vi "Apply Savitzky Golay Filter.vi"(0 "Waveform Graph":waveform(dbl)[](array[waveform])=[{"t0"=timestamp(0 s since 1904-01-01), "dt"=1.9999999999999998e-05, "Y"=array[781097 elements]}, {"t0"=timestamp(0 s since 1904-01-01), "dt"=1.9999999999999998e-05, "Y"=array[781097 elements]}], 2 "Savitzksky-Golay param":T1={"Sidepoints (M)"=20, "Filter Order"=5} {"Filter Order" scale=0.0..10.0; "Sidepoints (M)" scale=0.0..10.0}, 5 "error in (no error)":errorcluster) -> (14 "Waveform(s) out":waveform(dbl)[](array[waveform]), 19 "error out":errorcluster)   [LabVIEW 2019, in "Fcurve.lvclass"]
doc: "Decimates a waveform ptbypt with given parameters. Sidepoint (M), ordered polynomial refers to the polynomial order fitting parameter. \nNote: # of channels set to 1, can be configured to filter all channels when needed\n\nInput:\nWaveform graphs: [0] Deflection (V), [1] Zposition (V)\n\nOutput: \nWfms ([0] deflection) : [0] Filtered_Deflection (V). [1] Zposition (V)"
uses:
  Fcurve.lvclass
  <vilib>/ptbypt/NI_PtbyPt.lvlib
panel:
  out "Wfms ([0]deflection)":dbl[][](array[numeric])
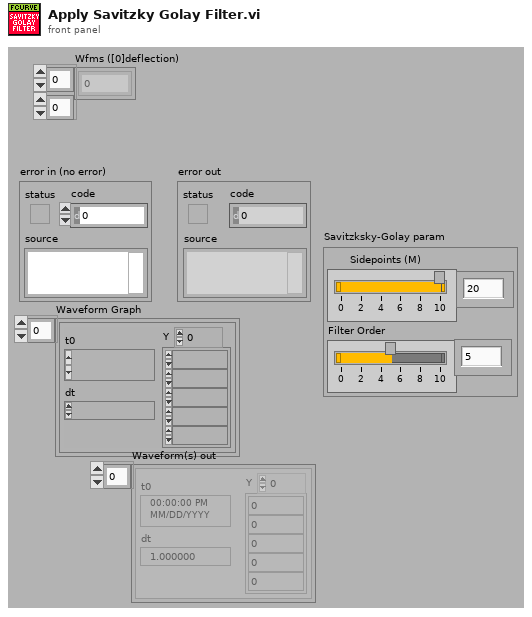
[diagram p1: front panel]
types:
  T1 = cluster{"Sidepoints (M)":i32, "Filter Order":i32}
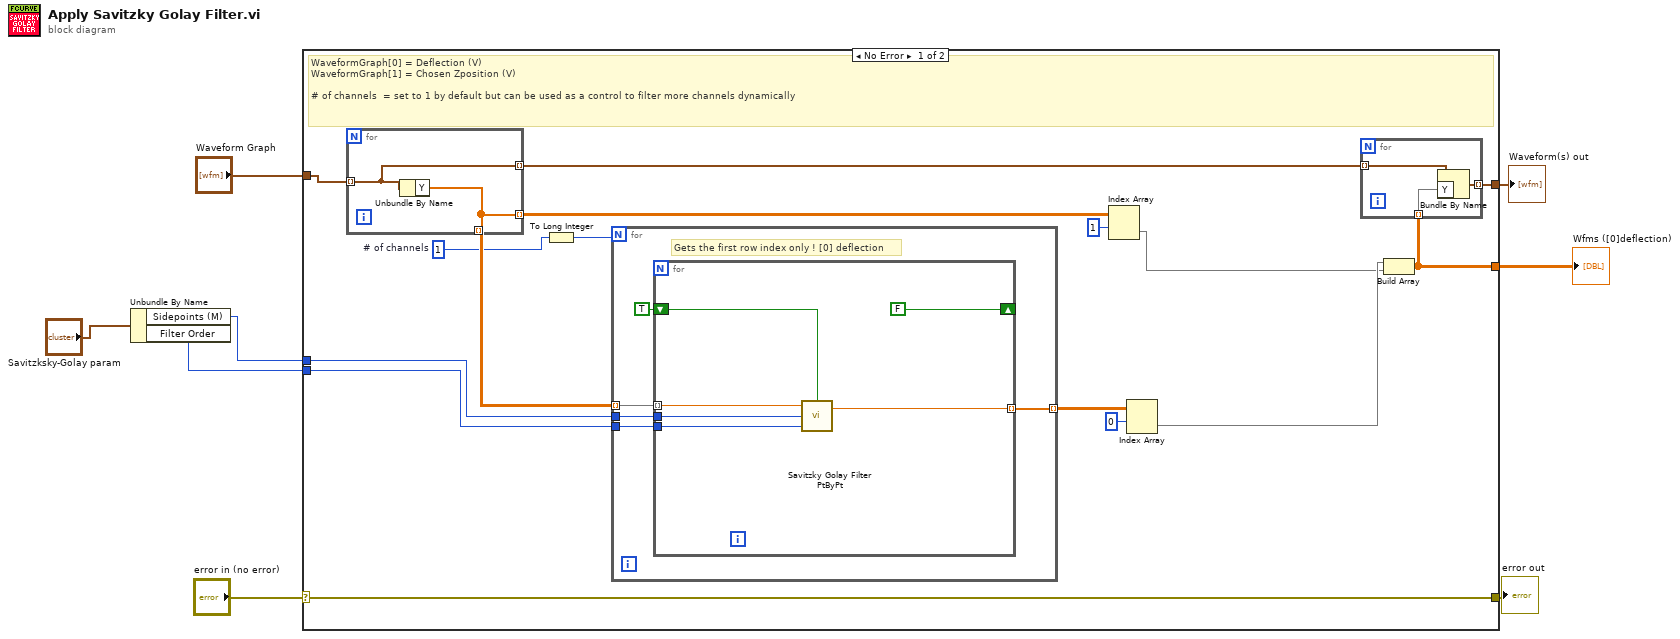
[diagram p0: block diagram]
diagram:
  n1 = Unbundle By Name("Savitzksky-Golay param") -> ("Sidepoints (M)"=w2:i32, "Filter Order"=w1:i32)
  n2 = case shown="No Error" "error in (no error)" {
    selector: "error in (no error)" -> [w24 w42]
    tunnel: [w24 w42] -> w7
    tunnel: w1 -> [w23 _]
    tunnel: w2 -> [w22 _]
    tunnel: "Waveform Graph" -> [w21 w41]
    tunnel: [w10 _] -> w5
    tunnel: [w9 w41] -> w4
    frame No Error {
      w16 = u8 1  # # of channels
      # "WaveformGraph[0] = Deflection (V)\nWaveformGraph[1] = Chosen Zposition (V)\n\n# of channels  = set to 1 by default but can be used as a control to filter more channels dynamically"
      n3 = for {
        tunnel: w21 -> [w39] mode=indexing
        tunnel: [w40] -> w20 mode=indexing
        tunnel: [w40] -> w19 mode=indexing
        tunnel: [w39] -> w11 mode=indexing
        n4 = Unbundle By Name(w39) -> ("Y"=w40:dbl[])
      }
      n5 = To Long Integer(number=w16) -> (32bit integer=w12:i32)
      n6 = for {
        N: w12 -> [_]
        tunnel: w23 -> [w31]
        tunnel: w22 -> [w30]
        tunnel: w20 -> [w29] mode=indexing
        tunnel: [w28] -> w17 mode=indexing
        # "Gets the first row index only ! [0] deflection"
        n7 = for {
          shift-right: [FALSE ("initialize")] -> _
          shift-left: TRUE ("initialize") -> [w38]
          tunnel: w30 -> [w36]
          tunnel: w31 -> [w35]
          tunnel: [w34] -> w28 mode=indexing
          tunnel: w29 -> [w33] mode=indexing
          n8 = call <vilib>:"Savitzky Golay Filter PtByPt.vi"("initialize"=w38, "order polynomial"=w35, "side points"=w36, "x"=w33) -> ("Filtered x"=w34:dbl)  [unwired: 1 out]
        }
      }
      n9 = Index Array(array=w19, index (row)=1) -> (element=w13:dbl[])  [unwired: 1 in]
      n10 = Index Array(array=w17, index (row)=0) -> (element=w14:dbl[])  [unwired: 1 in]
      n11 = Build Array(w14, w13) -> (w10:dbl[][])
      n12 = for {
        tunnel: w11 -> [w27] mode=indexing
        tunnel: w10 -> [w26] mode=indexing
        tunnel: [w25] -> w9 mode=indexing
        n13 = Bundle By Name(cluster=w27, "Y"=w26) -> (w25:waveform(dbl))
      }
    }
    frame Error {
    }
  }
  "error out" <- w7
  "Wfms ([0]deflection)" <- w5
  "Waveform(s) out" <- w4
